vi "set_caen_channelnames.vi"() -> ()   [LabVIEW 2018]
uses:
  channel_cluster.ctl
  <vilib>/Instr/_visa.llb/VISA Configure Serial Port (Instr).vi
  <vilib>/Utility/file.llb/Read Delimited Spreadsheet (string).vi
panel:
  out "concatenated string":string
  out "error out":errorcluster
  out "Display string":string
  in  "CAEN Serial Port":i32=6
  in  "Channel Settings File":path=path "C:/Users/User/Documents/Logs/Channel_Settings.csv"
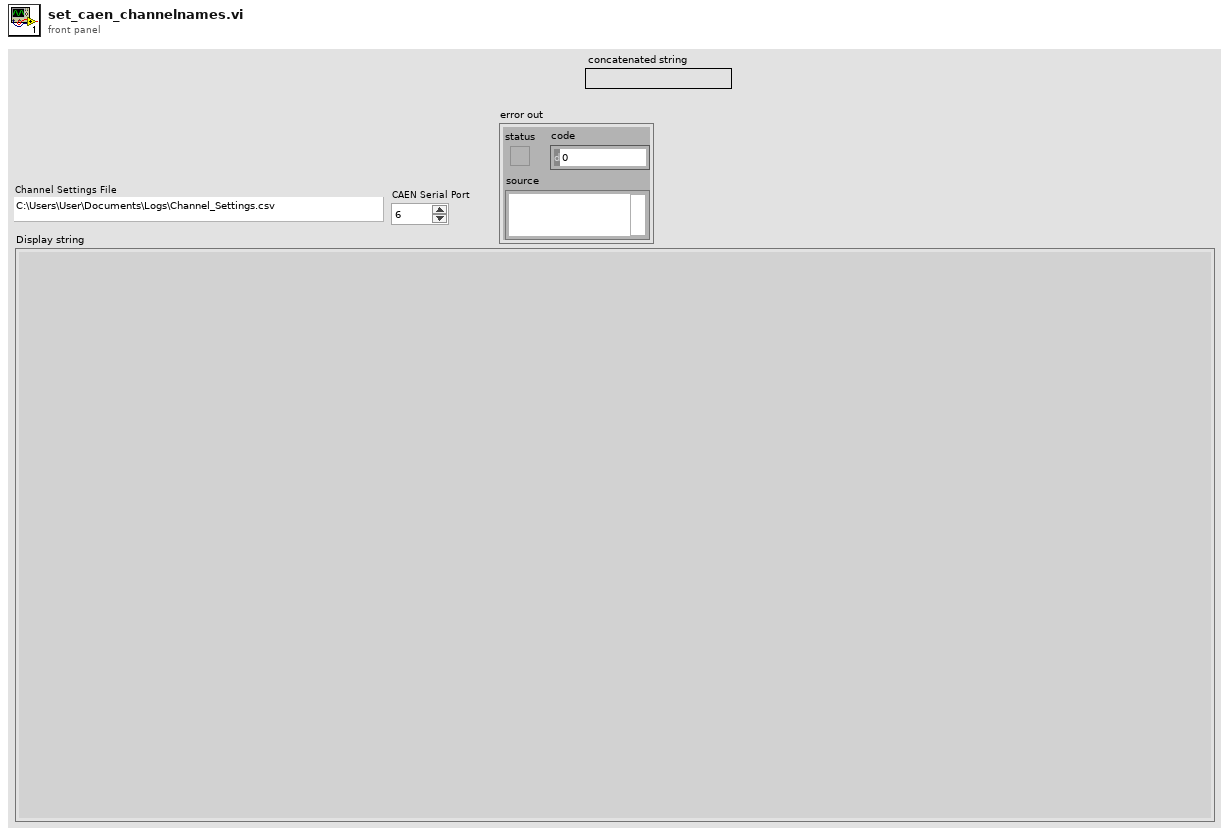
[diagram p1: front panel]
types:
  T1 = typedef "channel_cluster.ctl" = cluster{"Channel Name":string, "Crate":i32, "Card Type":string, "Card":i32, "Channel":i32, "Status Icon":picture, "Vmon (V)":dbl, "Vset (V)":dbl, "Imon (A)":dbl, "Iset (A)":dbl, "Timestamp":string, "ON/OFF":bool, "Status":string, "Vswmax (V)":dbl, "Flag":bool, "Vfile (V)":dbl, "Error Logged":bool[], "enable_file":bool}
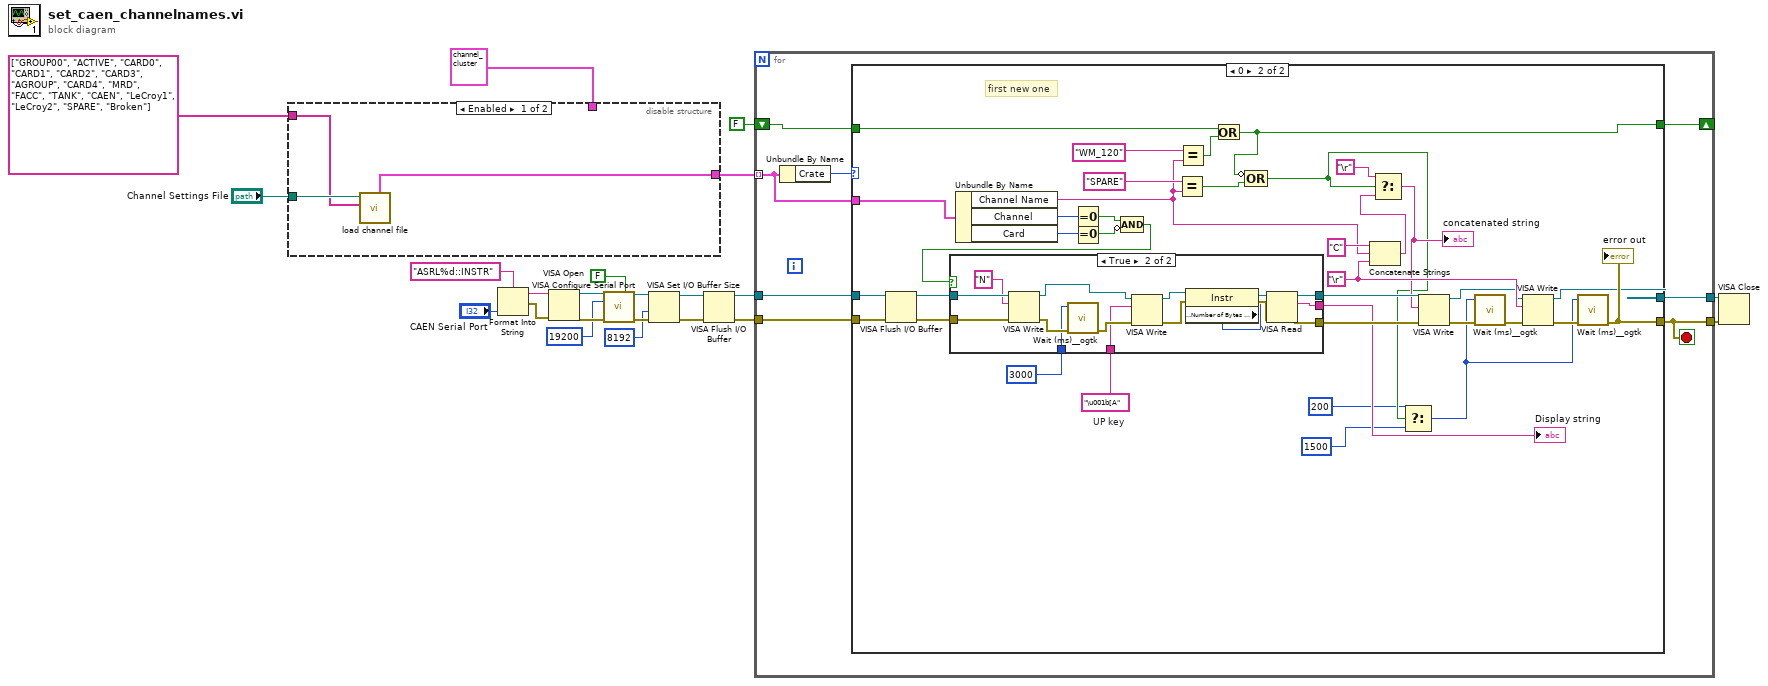
[diagram p0: block diagram]
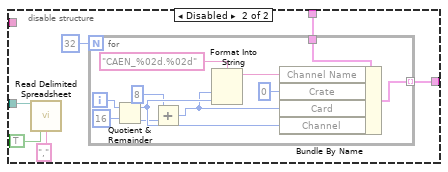
[diagram p2: hidden frame]
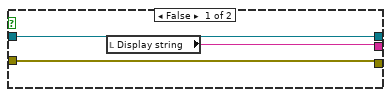
[diagram p4: hidden frame]
diagram:
  n1 = disable-structure shown="Enabled" {
    disable-tunnel: "Channel Settings File" -> [w25 w30]
    disable-tunnel: T1 {"Channel Name"="", "Crate"=0, "Card Type"="", "Card"=0, "Channel"=0, "Status Icon"=bytes[0], "Vmon (V)"=0.0, "Vset (V)"=0.0, "Imon (A)"=0.0, "Iset (A)"=0.0, "Timestamp"="", "ON/OFF"=FALSE, "Status"="", "Vswmax (V)"=0.0, "Flag"=FALSE, "Vfile (V)"=0.0, "Error Logged"=[], "enable_file"=FALSE} ("Channel cluster") -> [_ w31]
    disable-tunnel: [w24 w26] -> w3
    disable-tunnel: string[] ["GROUP00", "ACTIVE", "CARD0", "CARD1", "CARD2", "CARD3", "AGROUP", "CARD4", "MRD", "FACC", "TANK", "CAEN", "LeCroy1", "LeCroy2", "SPARE", "Broken"] ("Group Names") -> [w23 _]
    frame Enabled {
      n2 = call "load channel file.vi"("Group Names"=w23, "Channel List"=w25) -> ("Array"=w24:T1[])  [unwired: 5 in, 4 out]
    }
    frame Disabled {
      n3 = call-poly <vilib>:"Read Delimited Spreadsheet.vi"("file path (dialog if empty)"=w30, "transpose? (F)"=TRUE, "delimiter (\\t)"="," ("delimiter (\\t)")) -> ()  [unwired: 7 in, 6 out]
      n4 = for {
        N: 32 -> [_]
        tunnel: w31 -> [w42]
        tunnel: [w35] -> w26 mode=indexing
        i -> [w40]
        n5 = Quotient & Remainder(x=w40, y=16) -> (x-y*floor(x/y)=w37:i32, floor(x/y)=w34:i32)
        n6 = Add(x=8, y=w34) -> (x+y=w33:i32)
        n7 = Format Into String(format string="CAEN_%02d.%02d", w33, w37) -> (resulting string=w38:string)  [unwired: 2 in, 1 out]
        n8 = Bundle By Name(cluster=w42, "Channel Name"=w38, "Crate"=0, "Card"=w33, "Channel"=w37) -> (w35:T1)
      }
    }
  }
  n9 = Format Into String(format string="ASRL%d::INSTR" ("write buffer"), "CAEN Serial Port") -> (resulting string=w14:string, error out=w17:errorcluster)  [unwired: 2 in]
  n10 = VISA Open(error in (no error)=w17, VISA resource name=w14) -> (VISA resource name=w21:refnum<visa-resource-name>, error out=w20:errorcluster)  [unwired: 3 in]
  n11 = call-poly "VISA Configure Serial Port"("VISA resource name"=w21, "Enable Termination\nChar (T)"=FALSE ("Enable Termination\nChar (T)"), "baud rate (9600)"=u32 19200, "error in (no error)"=w20) -> ("VISA resource name out"=w13:refnum<visa-resource-name>, "error out"=w12:errorcluster)  [unwired: 10 in]
  n12 = VISA Set I/O Buffer Size(VISA resource name=w13, size (4096)=u32 8192 ("baud rate (9600)"), error in (no error)=w12) -> (VISA resource name out=w8:refnum<visa-resource-name>, error out=w7:errorcluster)  [unwired: 1 in]
  n13 = VISA Flush I/O Buffer(VISA resource name=w8, error in (no error)=w7) -> (VISA resource name out=w9:refnum<visa-resource-name>, error out=w10:errorcluster)  [unwired: 1 in]
  n14 = for {
    tunnel: w10 -> [w50]
    tunnel: w9 -> [w49]
    tunnel: w3 -> [w46] mode=indexing
    tunnel: [w47] -> w5
    tunnel: [w43] -> w6
    shift-right: [w44] -> _
    shift-left: FALSE ("result") -> [w45]
    stop <- w43 stop-if-true
    n15 = Unbundle By Name(w46) -> ("Crate"=w48:i32)
    n16 = case shown="0" w48 {
      tunnel: w50 -> [w52 w57]
      tunnel: w49 -> [w53 w56]
      tunnel: w46 -> [_ w90]
      tunnel: [w53 w74] -> w47
      tunnel: [w52 w77] -> w43
      tunnel: w45 -> [w51 w65]
      tunnel: [w51 w64] -> w44
      frame Default {
      }
      frame 0 {
        w62 = "\u001b[A"  # UP key
        w80 = "\r"
        # "first new one"
        n17 = VISA Flush I/O Buffer(VISA resource name=w56, error in (no error)=w57) -> (VISA resource name out=w55:refnum<visa-resource-name>, error out=w54:errorcluster)  [unwired: 1 in]
        n18 = Unbundle By Name(w90) -> ("Channel Name"=w68:string, "Channel"=w87:i32, "Card"=w86:i32)
        n19 = Equal To 0?(x=w87) -> (x = 0?=w85:bool)
        n20 = Equal To 0?(x=w86) -> (x = 0?=w84:bool)
        n21 = Compound Arithmetic op=AND(w85, invert w84) -> (w78:bool)
        n22 = case shown="True" w78 {
          tunnel: w54 -> [w92 w109]
          tunnel: w55 -> [w93 w108]
          tunnel: [w93 w106] -> w89
          tunnel: [w92 w105] -> w88
          tunnel: [w91 w104] -> w76
          tunnel: u32 3000 ("milliseconds to wait") -> [_ w99]
          tunnel: w62 -> [_ w94]
          frame False {
            n23 = local read "Display string"() -> (w91:string)
          }
          frame True {
            n24 = VISA Write(VISA resource name=w108, write buffer="N", error in (no error)=w109) -> (VISA resource name out=w97:refnum<visa-resource-name>, error out=w100:errorcluster)  [unwired: 1 out]
            n25 = call <userlib>:"Wait (ms)__ogtk.vi"("error in (no error)"=w100, "milliseconds to wait"=w99) -> ("error out"=w98:errorcluster)  [unwired: 8 in, 1 out]
            n26 = VISA Write(VISA resource name=w97, write buffer=w94, error in (no error)=w98) -> (VISA resource name out=w96:refnum<visa-resource-name>, error out=w95:errorcluster)  [unwired: 1 out]
            n27 = property class="Instr"(reference=w96, error in=w95) -> (reference out=w103:refnum<visa-resource-name>, error out=w102:errorcluster, "Serial Settings:Number of Bytes at Serial Port"=w101:u32)
            n28 = VISA Read(VISA resource name=w103, byte count=w101, error in (no error)=w102) -> (VISA resource name out=w106:refnum<visa-resource-name>, read buffer=w104:string, error out=w105:errorcluster)  [unwired: 1 out]
          }
        }
        "Display string" <- w76
        n29 = Equal?(x="SPARE", y=w68) -> (x = y?=w63:bool)
        n30 = Equal?(x="WM_120", y=w68) -> (x = y?=w66:bool)
        n31 = Or(x=w65, y=w66) -> (x .or. y?=w64:bool)
        n32 = Compound Arithmetic op=OR(invert w64, w63) -> (w61:bool)
        n33 = Concatenate Strings("C" ("write buffer"), w68, w80) -> (w70:string)
        n34 = Select(t="\r", s=w61, f=w70) -> (s? t:f=w69:string)
        "concatenated string" <- w69
        n35 = Select(t=u32 200 ("milliseconds to wait"), s=w61, f=u32 1500 ("milliseconds to wait")) -> (s? t:f=w58:u32)
        n36 = VISA Write(VISA resource name=w89, write buffer=w69, error in (no error)=w88) -> (VISA resource name out=w75:refnum<visa-resource-name>, error out=w82:errorcluster)  [unwired: 1 out]
        n37 = call <userlib>:"Wait (ms)__ogtk.vi"("error in (no error)"=w82, "milliseconds to wait"=w58) -> ("error out"=w81:errorcluster)  [unwired: 8 in, 1 out]
        n38 = VISA Write(VISA resource name=w75, write buffer=w80, error in (no error)=w81) -> (VISA resource name out=w74:refnum<visa-resource-name>, error out=w79:errorcluster)  [unwired: 1 out]
        n39 = call <userlib>:"Wait (ms)__ogtk.vi"("error in (no error)"=w79, "milliseconds to wait"=w58) -> ("error out"=w77:errorcluster)  [unwired: 8 in, 1 out]
        "error out" <- w77
      }
    }
  }
  n40 = VISA Close(VISA resource name=w5, error in (no error)=w6) -> ()  [unwired: 1 out]
